vi "tsapp_disconnect_win32.vi"(8 "错误输入（无错误）":errorcluster) -> (0 "错误输出":errorcluster, 1 "tsapp_disconnect":i32, 2 "DisConnectSeccessfully":bool)   [LabVIEW 2016]
uses:
  TSMaster.dll
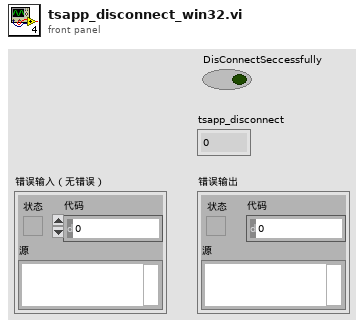
[diagram p1: front panel]
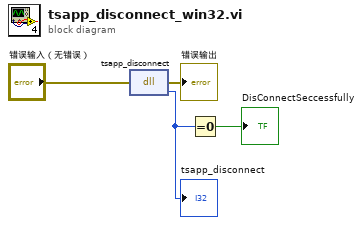
[diagram p0: block diagram]
diagram:
  n1 = dll-call lib="C:/Users/Eric/Desktop/LabVIEW/TSMasterAPI/Win32/CANopen_TS_2015/TSMaster.dll" fn="tsapp_disconnect"(error in="错误输入（无错误）") -> (error out=→"错误输出":errorcluster, "tsapp_disconnect"=w1:i32)  [unwired: 2 in, 1 out]
  "tsapp_disconnect" <- w1
  n2 = Equal To 0?(x=w1) -> (x = 0?=→"DisConnectSeccessfully":bool)
